vi "移动鼠标往下LV8.6.vi"   [LabVIEW 2017]
uses:
  user32.dll
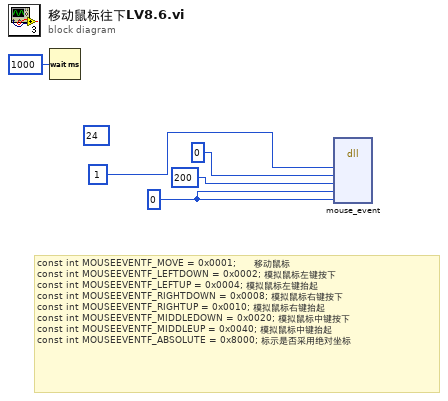
[diagram p0: block diagram]
diagram:
  w5 = 0 ("dx")
  (unwired) 24 ("dwFlags")
  # "const int MOUSEEVENTF_MOVE = 0x0001;      移动鼠标 \nconst int MOUSEEVENTF_LEFTDOWN = 0x0002; 模拟鼠标左键按下 \nconst int MOUSEEVENTF_LEFTUP = 0x0004; 模拟鼠标左键抬起 \nconst int MOUSEEVENTF_RIGHTDOWN = 0x0008; 模拟鼠标右键按下 \nconst int MOUSEEVENTF_RIGHTUP = 0x0010; 模拟鼠标右键抬起 \nconst int MOUSEEVENTF_MIDDLEDOWN = 0x0020; 模拟鼠标中键按下 \nconst int MOUSEEVENTF_MIDDLEUP = 0x0040; 模拟鼠标中键抬起 \nconst int MOUSEEVENTF_ABSOLUTE = 0x8000; 标示是否采用绝对坐标"
  n1 = Wait (ms)(milliseconds to wait=u32 1000 ("等待时间（毫秒）")) -> ()  [unwired: 1 out]
  n2 = dll-call lib="user32.dll" fn="mouse_event"("dwFlags"=1, "dx"=0, "dy"=200, "cButtons"=w5, "dwExtraInfo"=w5) -> ()  [unwired: 9 in, 2 out]
